vi "PicoScope4000GetValues.vi"(5 "Segment Range":T1 {"toSegmentIndex" format="%.4p"; "fromSegmentIndex" format="%.4p"}, 7 "Buffer and Transfer Settings":T2 {"Down-Sample Mode" items=["None", "Aggregate", "Average"]; "Down Sample Ratio" step=1; "Samples" format="%_6p"}, 8 "error in (no error)":errorcluster, 11 "handle in":i16) -> (0 "error out":errorcluster, 3 "handle out":i16, 4 "overflow":i16 format="%04b", 6 "noOfSamples":u64)   [LabVIEW 2009]
doc: "Calls GetValuesOverlapped"
uses:
  ps4000.dll
  shared/Segment Range.ctl
  PicoScope4000Buffer and Transfer Settings.ctl
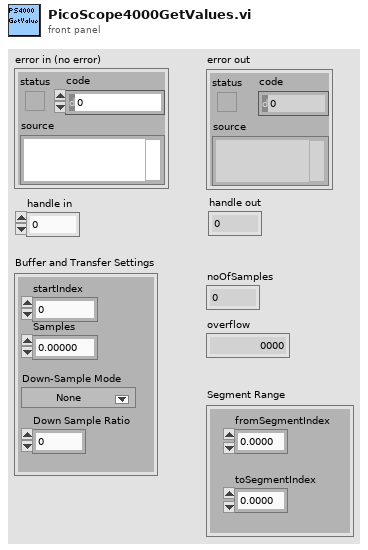
[diagram p1: front panel]
types:
  T1 = typedef "Segment Range.ctl" = cluster{"fromSegmentIndex":u64, "toSegmentIndex":u64}
  T2 = typedef "PicoScope4000Buffer and Transfer Settings.ctl" = cluster{"startIndex":u64, "Samples":u64, "Down Sample Ratio":u64, "Down-Sample Mode":u32}
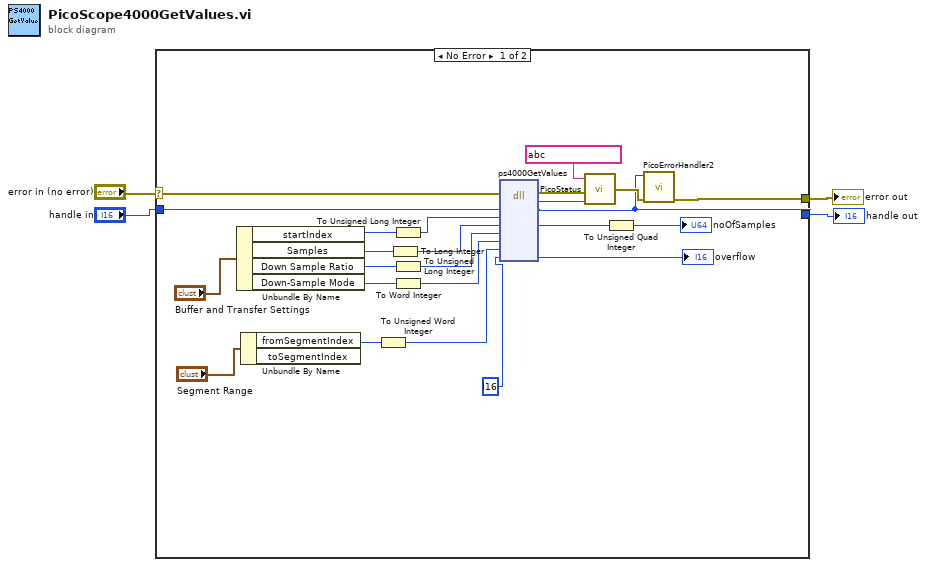
[diagram p0: block diagram]
diagram:
  n1 = case shown="No Error" "error in (no error)" {
    selector: "error in (no error)" -> [w12 w29]
    tunnel: "handle in" -> [w13 w30]
    tunnel: [w10 w30] -> w4
    tunnel: [w25 w29] -> w3
    frame #0 {
      n2 = Unbundle By Name("Buffer and Transfer Settings") -> ("startIndex"=w22:u64, "Samples"=w20:u64, "Down Sample Ratio"=w21:u64, "Down-Sample Mode"=w6:u32)
      n3 = Unbundle By Name("Segment Range") -> ("fromSegmentIndex"=w23:u64)  [unwired: 1 out]
      n4 = To Unsigned Word Integer(number=w23) -> (unsigned 16bit integer=w17:u16)
      n5 = To Long Integer(number=w20) -> (32bit integer=w15:i32)
      n6 = To Unsigned Long Integer(number=w22) -> (unsigned 32bit integer=w14:u32)
      n7 = To Unsigned Long Integer(number=w21) -> (unsigned 32bit integer=w16:u32)
      n8 = To Word Integer(number=w6) -> (16bit integer=w5:i16)
      n9 = dll-call lib="PS4000.dll" fn="ps4000GetValues" ("ps3000.dll:_ps3000_open_unit@0")(error in=w12, "handle"=w13, "startIndex"=w14, "noOfSamples"=w15, "downSampleRatio"=w16, "downSampleRatioMode"=w5, "segmentIndex"=w17, "overflow"=i16 ?) -> (error out=w11:errorcluster, "PICO_STATUS"=w9:u32, "handle"=w10:i16, "noOfSamples"=w8:i32, "overflow"=→"overflow":i16)  [unwired: 6 in, 1 out]
      n10 = call "PicoStatus.vi"("PICO STATUS"=w9, "error in"=w11, "source"=string ?) -> ("error out"=w28:errorcluster)
      n11 = To Unsigned Quad Integer(1:w8) -> (0:→"noOfSamples":u64)
      n12 = call "PicoErrorHandler2.vi"("error in (no error)"=w28, "handle In"=w10) -> ("error out"=w25:errorcluster)  [unwired: 9 in]
    }
    frame #1 {
    }
  }
  "error out" <- w3
  "handle out" <- w4
